vi "FGV.vi"(8 "error in":errorcluster, 10 "Action":enum16{"Create", "Fire", "Get", "Destroy"}(ring)=enum."Destroy") -> (0 "error out":errorcluster)   [LabVIEW 2018]
panel:
  in  "Queue name":string
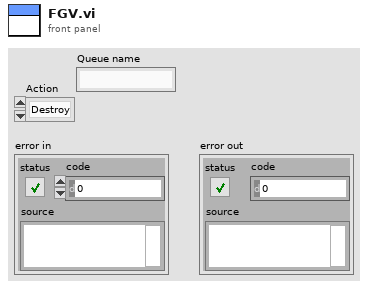
[diagram p1: front panel]
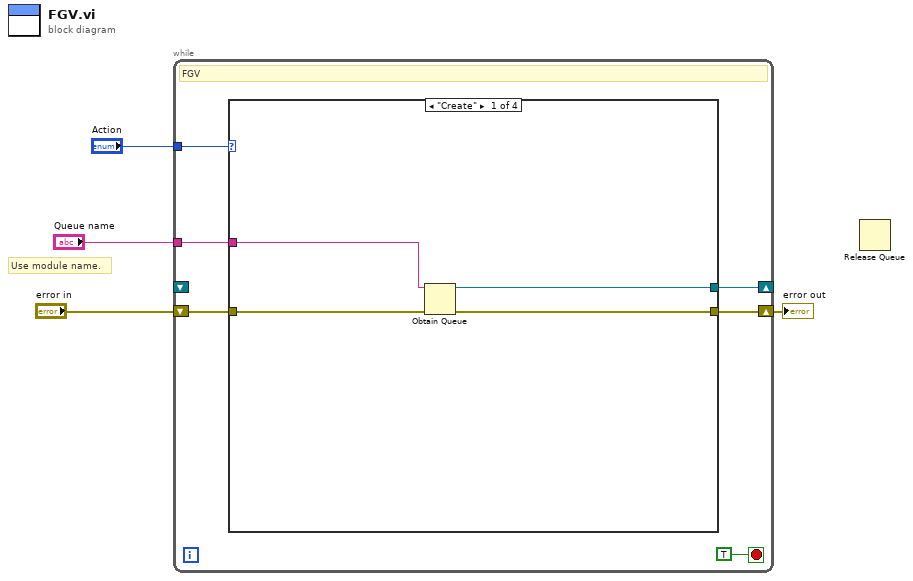
[diagram p0: block diagram]
diagram:
  # "Use module name."
  n1 = while {
    tunnel: "Action" -> [w9]
    shift-right: [w8] -> _
    shift-left: _ -> [_]
    shift-right: [w7] -> w3
    shift-left: "error in" -> [w6]
    tunnel: "Queue name" -> [w5]
    stop <- TRUE stop-if-true
    # "FGV"
    n2 = case shown="\"Create\"" w9 {
      tunnel: [w14 _ _ _] -> w8
      tunnel: [w13 _ _ _] -> w7
      tunnel: w6 -> [w12 _ _ _]
      tunnel: w5 -> [w11 _ _ _]
      frame "Create" {
        n3 = Obtain Queue(name (unnamed)=w11, error in (no error)=w12) -> (queue out=w14:refnum<queue>, error out=w13:errorcluster)  [unwired: 3 in, 1 out]
      }
      frame "Fire" {
      }
      frame "Get", Default {
      }
      frame "Destroy" {
      }
    }
  }
  "error out" <- w3
  n4 = Release Queue() -> ()  [unwired: 3 in, 3 out]
